vi "Thorlabs_SC10_OpenOrClose.vi"(8 "error in (no error)":errorcluster, 11 "Input string":string="ens\r> ens?\r0\r> ") -> (0 "error out":errorcluster, 3 "Open?":bool)   [LabVIEW 2022 SP3]
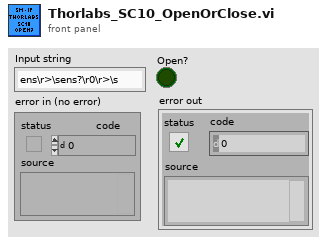
[diagram p1: front panel]
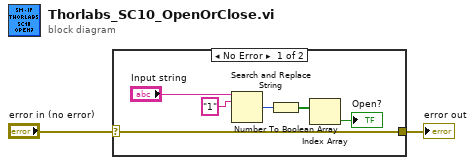
[diagram p0: block diagram]
diagram:
  n1 = case shown="No Error" "error in (no error)" {
    selector: "error in (no error)" -> [w3 w9]
    tunnel: [w3 w9] -> w1
    frame No Error {
      n2 = Search and Replace String(input string="Input string", search string="1") -> (number of replacements=w6:i32)  [unwired: 6 in, 3 out]
      n3 = Number To Boolean Array(number=w6) -> (Boolean array=w5:bool[])
      n4 = Index Array(array=w5) -> (element=→"Open?":bool)  [unwired: 1 in]
    }
    frame Error {
    }
  }
  "error out" <- w1
